vi "getPolarity.vi"(0 "PMX4CXSAController in":refnum<class "PMX4CXSAController.lvclass">, 2 "axis (in) - nc; for this device polarity items are not axis-specific":T1, 5 "error in (no error)":errorcluster) -> (14 "PMX4CXSAController out":refnum<class "PMX4CXSAController.lvclass">, 16 "polarity_items (out)":T2[](array[typedef]), 19 "error out":errorcluster)   [LabVIEW 2013, in "classes.lvlib" / "PMX4CXSAController.lvclass"]
doc: "Produced By:\n\n<B>Kod Integrations, LLC</B>\n4835 Marianne Drive\nMount Airy, MD 21771\nhttp://www.kodintegrations.com\nemail: info@kodintegrations.com\nphone: (240) 687-1288"
uses:
  PMX4CXSAController.lvclass
  polarity_item.ctl
  polarity.ctl
  axis.ctl
  simple_actions.ctl
  _Controller.lvclass
  common.lvlib
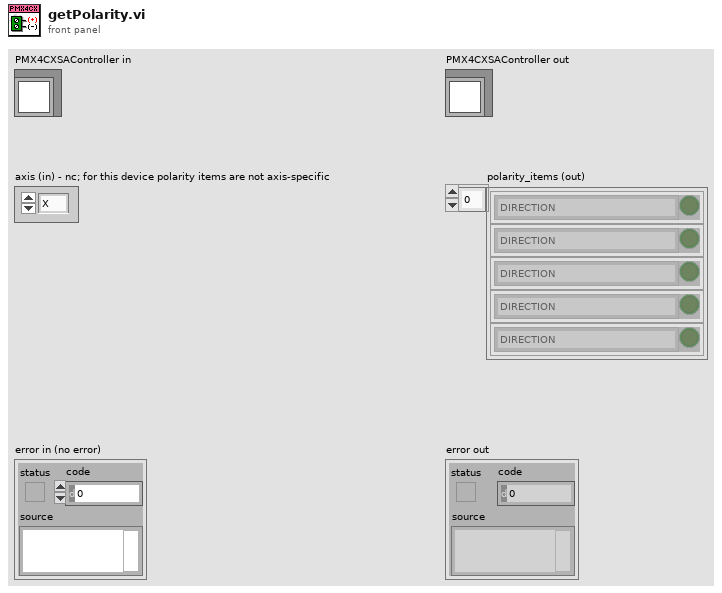
[diagram p1: front panel]
types:
  T1 = typedef "common.lvlib/axis.ctl" = enum16{"X", "Y", "Z", "U"}
  T2 = typedef "common.lvlib/polarity_item.ctl" = cluster{"item":T3, "status":bool}
  T3 = typedef "common.lvlib/polarity.ctl" = enum16{"DIRECTION", "LIMIT", "HOME", "DIG_OUT", "DIG_IN", "ENABLE_OUT", "JUMP_ERR", "LATCH", "Z-CHAN_INDEX", "ENCODER_DECODING:1X", "ENCODER_DECODING:2X", "ENCODER_DECODING:4X", "ALARM", "STANDALONE_ERR", "-", "<reserved/nc>"}
  T4 = typedef "common.lvlib/simple_actions.ctl" = enum16{"from_value", "to_value"}
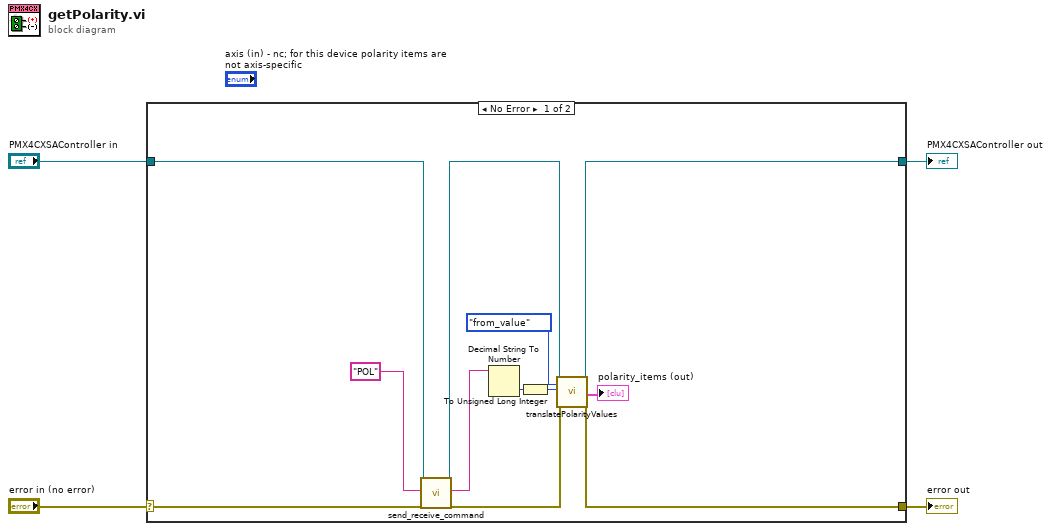
[diagram p0: block diagram]
diagram:
  n1 = case shown="No Error" "error in (no error)" {
    selector: "error in (no error)" -> [w10 w18]
    tunnel: [w9 w18] -> w3
    tunnel: [w6 w17] -> w1
    tunnel: "PMX4CXSAController in" -> [w8 w17]
    frame No Error {
      n2 = call "send_receive_command.vi"("reference (in)"=w8, "ASCII Command (in)"="POL", "error in (no error)"=w10) -> ("reference (out)"=w7:refnum<class "PMX4CXSAController.lvclass">, "response (out)"=w16:string, "error out"=w11:errorcluster)  [unwired: 12 in, 2 out]
      n3 = Decimal String To Number(string=w16) -> (number=w14:i32)  [unwired: 2 in, 1 out]
      n4 = To Unsigned Long Integer(number=w14) -> (unsigned 32bit integer=w12:u32)
      n5 = call-dynamic "translatePolarityValues.vi"("PMX4CXSAController in"=w7, "simple_actions"=simple_actions."from_value", "polarity_value (in)"=w12, "error in (no error)"=w11) -> ("PMX4CXSAController out"=w6:refnum<class "PMX4CXSAController.lvclass">, "polarity_items (out)"=→"polarity_items (out)":T2[], "error out"=w9:errorcluster)  [unwired: 12 in, 1 out]
    }
    frame Error {
    }
  }
  "error out" <- w3
  "PMX4CXSAController out" <- w1
